vi "LM model function orbit multi magnetometer.vi"(3 "output control":T1, 4 "data":variant, 5 "X":dbl[](array[numeric]), 6 "a":dbl[](array[numeric])) -> (0 "error out":errorcluster, 1 "f'(X,a)":dbl[][](array[numeric]), 2 "f(X,a)":dbl[](array[numeric]))   [LabVIEW 2017]
doc: "This template is the starting point for creating a model function to be passed to the Nonlinear Curve Fit.vi."
uses:
  <vilib>/gmath/NumericalOptimization/LM_output select.ctl
  typedefs/orbit magnetic field data.ctl
  typedefs/magnetomter reading set.ctl
  <vilib>/gmath/NI_Gmath.lvlib
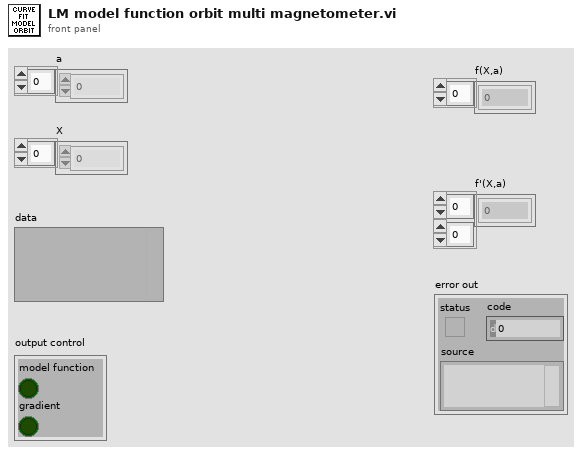
[diagram p1: front panel]
types:
  T1 = typedef "NI_Gmath.lvlib/LM_output select.ctl" = cluster{"model function":bool, "gradient":bool}
  T2 = typedef "orbit magnetic field data.ctl" = cluster{"magnetometer readings":T3[], "L":dbl, "omega":dbl, "t0":fxp<+,48,48>}
  T3 = typedef "magnetomter reading set.ctl" = cluster{"time":fxp<+,48,48>, "mag readings":cluster{"magnetometer index":dbl, "Bx":dbl, "By":dbl, "Bz":dbl, "magnetometer x":dbl, "magnetometer y":dbl}[]}
  T4 = cluster{"a[0]":dbl, "a[1]":dbl, "a[2]":dbl, "a[3]":dbl, "a[4]":dbl, "a[5]":dbl, "a[6]":dbl, "a[7]":dbl, "a[8]":dbl, "a[9]":dbl, "a[10]":dbl}
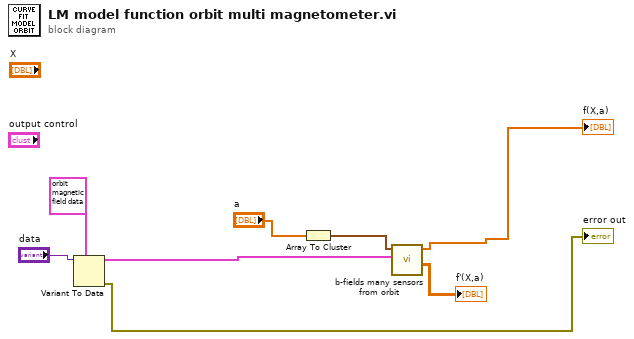
[diagram p0: block diagram]
diagram:
  n1 = Variant To Data(type=T2 {"magnetometer readings"=[], "L"=0.0, "omega"=0.0, "t0"=0.0} ("orbit magnetic field data"), Variant="data") -> (data=w3:T2, error out=→"error out":errorcluster)  [unwired: 1 in]
  n2 = Array To Cluster(array="a") -> (cluster=w4:T4)
  n3 = call "b-fields many sensors from orbit.vi"("orbit magnetic field data"=w3, "orbit parameters"=w4) -> ("derivatives"=→"f'(X,a)":dbl[][], "predicted field"=→"f(X,a)":dbl[])  [unwired: 4 in, 4 out]
